vi "Sample Client.vi"() -> ()   [LabVIEW 2021]
uses:
  CIF_PluginLoader_client/RPC Messages/cif_management_common_LoaderInfoFull.ctl
  CIF_PluginLoader_client/RPC Messages/cif_management_common_LoaderType.ctl
  CIF_PluginLoader_client/RPC Messages/cif_pluginloader_DiscoveredPlugin.ctl
  CIF_PluginLoader_client/RPC Messages/cif_common_Version.ctl
  CIF_PluginLoader_client/RPC Messages/cif_management_common_PluginMetadata.ctl
  CIF_Plugin_Loader_Client_Wrapper/CIFPluginLoaderClientWrapper.lvlib
  CIF_PluginLoader_client/CIF_PluginLoader_client.lvlib
panel:
  out "discovered_plugins":T1[](array[typedef])
  out "loader_info":T4
  out "error out":errorcluster
  in  "address":string="localhost:"
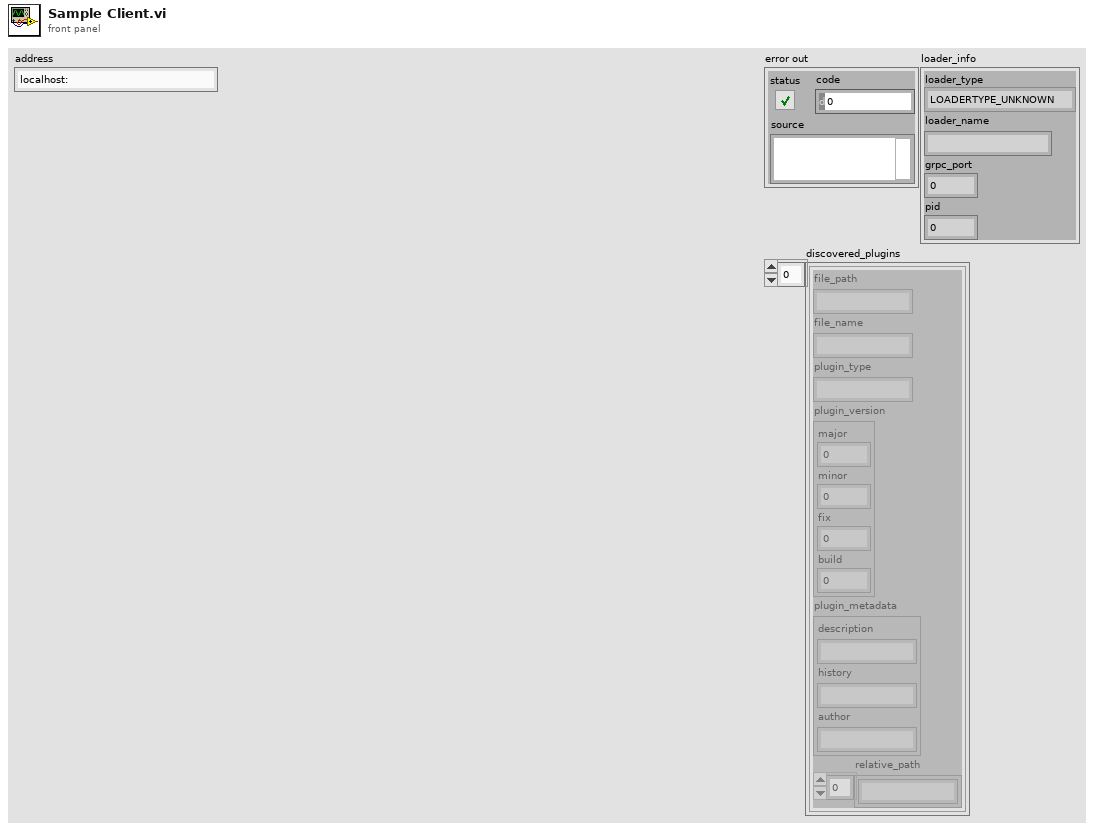
[diagram p1: front panel]
types:
  T1 = typedef "CIF_PluginLoader_client.lvlib/cif_pluginloader_DiscoveredPlugin.ctl" = cluster{"file_path":string, "file_name":string, "plugin_type":string, "plugin_version":T2, "plugin_metadata":T3, "relative_path":string[]}
  T2 = typedef "CIF_PluginLoader_client.lvlib/cif_common_Version.ctl" = cluster{"major":u32, "minor":u32, "fix":u32, "build":u32}
  T3 = typedef "CIF_PluginLoader_client.lvlib/cif_management_common_PluginMetadata.ctl" = cluster{"description":string, "history":string, "author":string}
  T4 = typedef "CIF_PluginLoader_client.lvlib/cif_management_common_LoaderInfoFull.ctl" = cluster{"loader_type":T5, "loader_name":string, "grpc_port":i32, "pid":u32}
  T5 = typedef "CIF_PluginLoader_client.lvlib/cif_management_common_LoaderType.ctl" = enum32{"LOADERTYPE_UNKNOWN", "LOADERTYPE_LABVIEW"}
  T6 = typedef "grpc-lvsupport-release.lvlib/grpcId.ctl" = u64
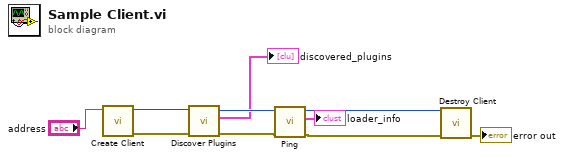
[diagram p0: block diagram]
diagram:
  n1 = call "Create Client.vi"("address"="address") -> ("error out"=w4:errorcluster, "gRPC ID Out"=w5:T6)  [unwired: 9 in]
  n2 = call "Discover Plugins.vi"("error in"=w4, "gRPC ID in"=w5) -> ("error out"=w3:errorcluster, "discovered_plugins"=→"discovered_plugins":T1[], "gRPC ID out"=w2:T6)  [unwired: 7 in]
  n3 = call "Ping.vi"("error in"=w3, "gRPC ID in"=w2) -> ("error out"=w9:errorcluster, "loader_info"=→"loader_info":T4, "gRPC ID out"=w10:T6)  [unwired: 7 in]
  n4 = call "Destroy Client.vi"("error in"=w9, "gRPC ID"=w10) -> ("error out"=→"error out":errorcluster)  [unwired: 9 in]
